vi "TrajFilter.vi"(6 "AnkleTraj_Init":bool, 9 "CurrentTraj":dbl[][](array[numeric])) -> (0 "AnkleTraj_Init 2":bool, 3 "AverageTraj":dbl[][](array[numeric]))   [LabVIEW 2015, in "ForceField.lvclass"]
uses:
  ForceField.lvclass
panel:
  in  "b":dbl[](array[numeric])=[1.0, 0.0, 0.1716]
  in  "a":dbl[](array[numeric])=[0.2929, 0.5858, 0.2929]
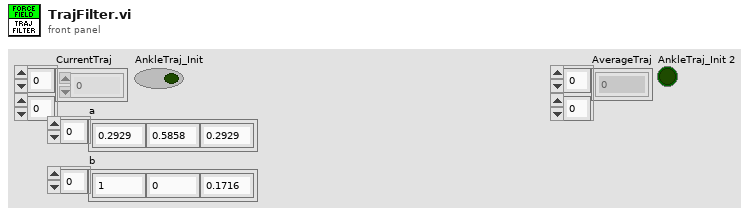
[diagram p1: front panel]
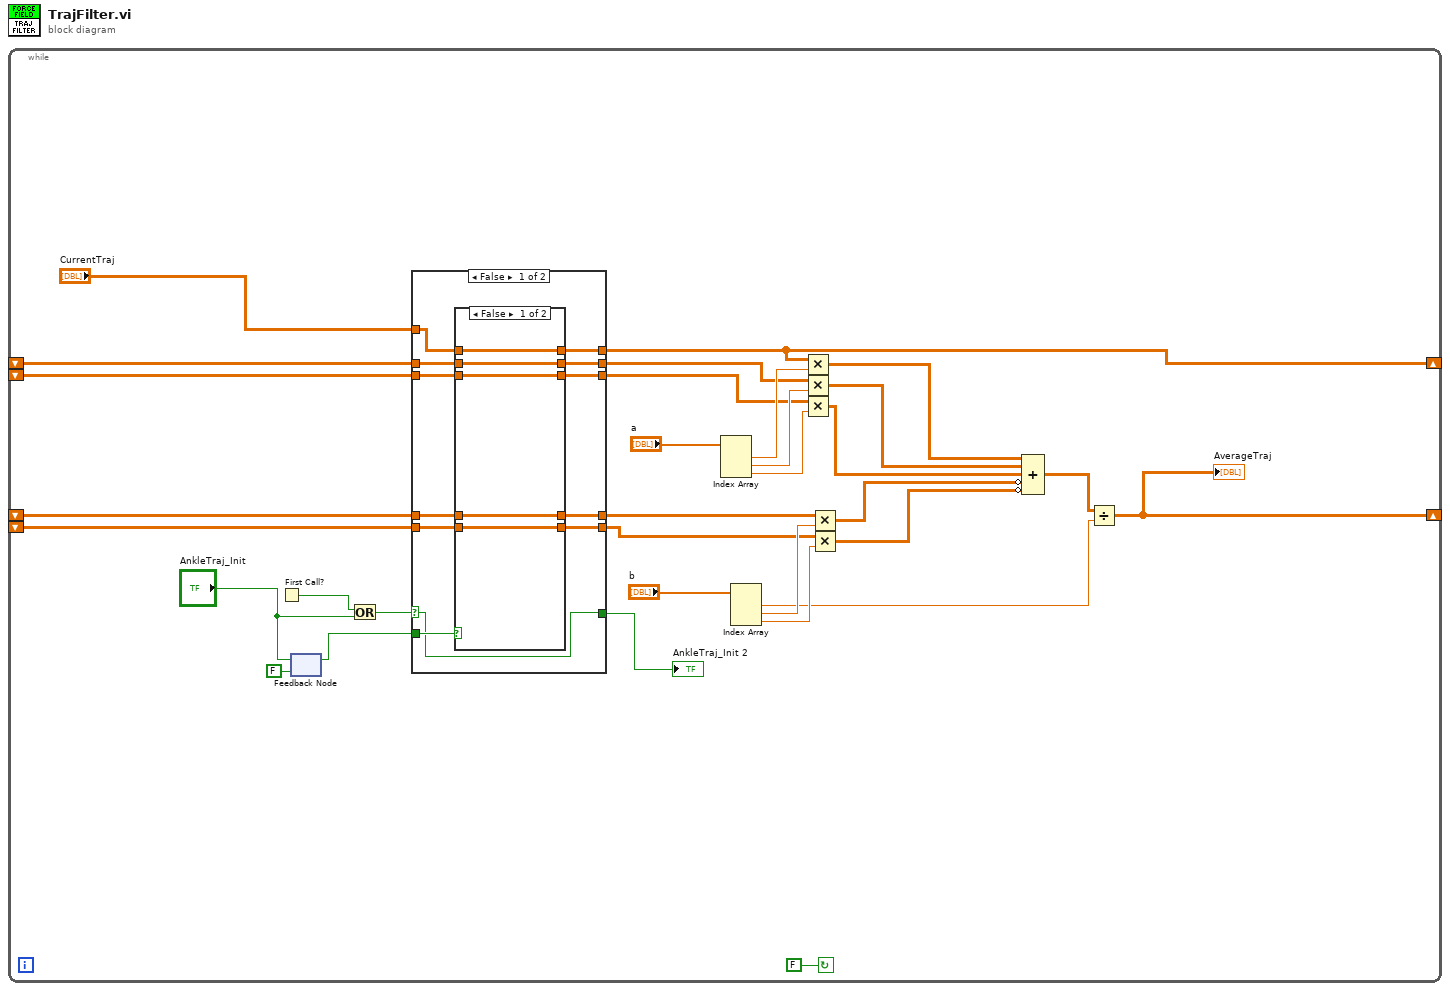
[diagram p0: block diagram]
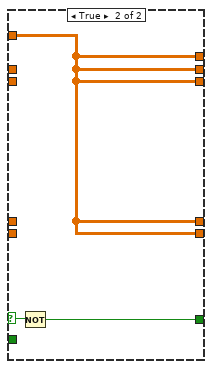
[diagram p3: hidden frame]
diagram:
  n1 = while {
    shift-right: [w30] -> _
    shift-left: _ -> [w15]
    shift-left: _ -> [w12]
    shift-right: [w17] -> _
    shift-left: _ -> [w10]
    shift-left: _ -> [w8]
    stop <- FALSE continue-if-true
    n2 = First Call?() -> (First Call?: T/F=w4:bool)
    n3 = feedback-in #1("AnkleTraj_Init") -> ()
    n4 = feedback #1(FALSE ("Init")) -> (w3:bool)
    n5 = Or(x=w4, y="AnkleTraj_Init") -> (x .or. y?=w6:bool)
    n6 = case shown="False" w6 {
      selector: w6 -> [w33 w54]
      tunnel: [w43 w55] -> w30
      tunnel: w15 -> [w42 _]
      tunnel: [w39 w55] -> w14
      tunnel: "CurrentTraj" -> [w44 w55]
      tunnel: w12 -> [w41 _]
      tunnel: [w40 w55] -> w11
      tunnel: w10 -> [w38 _]
      tunnel: [w37 w55] -> w9
      tunnel: w8 -> [w35 _]
      tunnel: [w36 w55] -> w7
      tunnel: w3 -> [w34 _]
      tunnel: [w33 w53] -> w1
      frame False {
        n7 = case shown="False" w34 {
          tunnel: w44 -> [w49 w52]
          tunnel: [w49 w52] -> w43
          tunnel: w42 -> [w47 w51]
          tunnel: w41 -> [w48 _]
          tunnel: [w48 w51] -> w40
          tunnel: [w47 w51] -> w39
          tunnel: w38 -> [w46 w50]
          tunnel: [w46 w50] -> w37
          tunnel: [w45 w50] -> w36
          tunnel: w35 -> [w45 _]
          frame False {
          }
          frame True {
          }
        }
      }
      frame True {
        n8 = Not(x=w54) -> (.not. x?=w53:bool)
      }
    }
    "AnkleTraj_Init 2" <- w1
    n9 = Index Array(array="a") -> (element #1=w29:dbl, element #2=w28:dbl, element #3=w27:dbl)  [unwired: 3 in]
    n10 = Index Array(array="b") -> (element #1=w16:dbl, element #2=w22:dbl, element #3=w21:dbl)  [unwired: 3 in]
    n11 = Multiply(x=w30, y=w29) -> (x*y=w26:dbl[][])
    n12 = Multiply(x=w14, y=w28) -> (x*y=w25:dbl[][])
    n13 = Multiply(x=w11, y=w27) -> (x*y=w24:dbl[][])
    n14 = Multiply(x=w9, y=w22) -> (x*y=w20:dbl[][])
    n15 = Multiply(x=w7, y=w21) -> (x*y=w19:dbl[][])
    n16 = Compound Arithmetic op=ADD(w26, w25, w24, invert w20, invert w19) -> (w18:dbl[][])
    n17 = Divide(x=w18, y=w16) -> (x/y=w17:dbl[][])
    "AverageTraj" <- w17
  }
